vi "Teleop.vi"   [LabVIEW 2013]
uses:
  Robot/Logical Systems/Drive Train/Drive Train Commands/Drive By Power/Drive by Power Class/Drive by Power.lvclass
  Robot/Robot Actors/System Actor/System Actor Messages/Start Command Msg/Start Command Msg.lvclass/Start Command Msg.ctl
  <vilib>/ActorFramework/Message Enqueuer/Message Enqueuer.lvclass/Message Enqueuer.ctl
  <vilib>/ActorFramework/Message Enqueuer/Enqueue.vi
  Robot Global.vi
  <vilib>/ActorFramework/Message Priority Queue/Priority Enqueue.vi
  Robot/Robot Actors/System Actor/System Actor Messages/Start Command Msg/Start Command Msg.lvclass
  Robot/Logical Systems/Driver/Driver-Logical Messages/New Driver Input Msg/New Driver Input Msg.lvclass
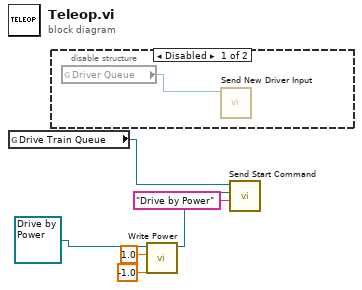
[diagram p0: block diagram]
diagram:
  n1 = global read "Robot Global.vi" "Drive Train Queue"() -> (w3:refnum<class "Message Enqueuer.lvclass">)
  n2 = disable-structure shown="Disabled" {
    frame Disabled {
      n3 = global read "Robot Global.vi" "Driver Queue"() -> (w7:refnum<class "Message Enqueuer.lvclass">)
      n4 = call "Send New Driver Input.vi"("Message Enqueuer"=w7) -> ()  [unwired: 9 in, 2 out]
    }
    frame Enabled {
    }
  }
  n5 = call-dynamic "Write Power.vi"("Right Power"=-1.0, "Left Power"=1.0, "Drive by Power in"=refnum<class "Drive by Power.lvclass"> refnum ("Logical Systems.lvlib:Drive Train.lvlib:Drive by Power.lvlib:Drive by Power.lvclass")) -> ("Drive by Power out"=w2:refnum<class "Drive by Power.lvclass">)  [unwired: 7 in, 1 out]
  n6 = call "Send Start Command.vi"("Command Name"="Drive by Power", "Robot Actors.lvlib:Command.lvlib:Command.lvclass"=w2, "Message Enqueuer"=w3) -> ()  [unwired: 7 in, 2 out]
